vi "FTW-Endpoint-Tell.vi"(0 "FTW Socket":refnum<class "FTW-Endpoint.lvclass">, 5 "Message Header":string, 7 "Message Body":string, 9 "Timeout":i32 format="%dmsec", 11 "error in":errorcluster) -> (4 "FTW Socket out":refnum<class "FTW-Endpoint.lvclass">, 6 "Timed out?":bool, 15 "error out":errorcluster)   [LabVIEW 2012, in "FTW-Actor.lvlib" / "FTW-Endpoint.lvclass"]
uses:
  FTW-Endpoint.lvclass
  Request/FTW-Request.lvclass
panel:
  # "Inputs"
  # "Outputs"
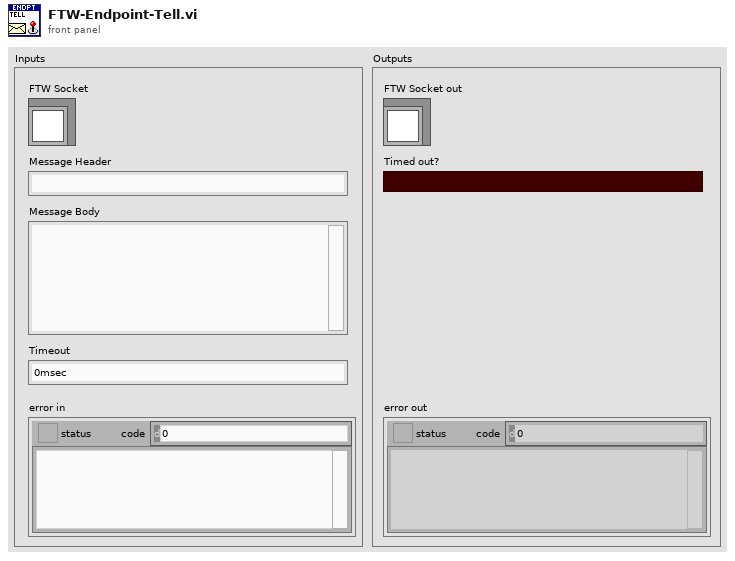
[diagram p1: front panel]
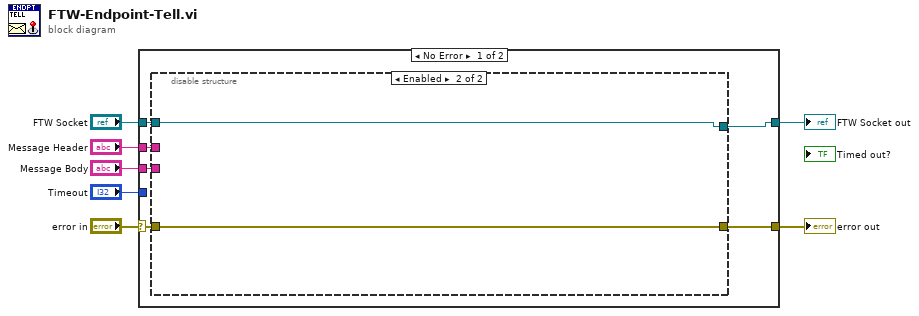
[diagram p0: block diagram]
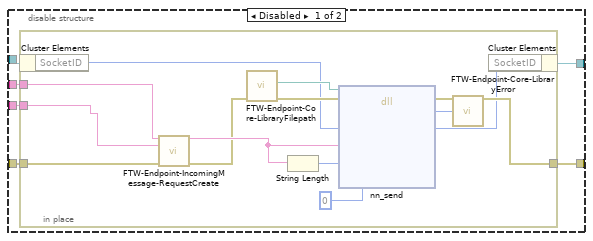
[diagram p2: hidden frame]
diagram:
  n1 = case shown="No Error" "error in" {
    selector: "error in" -> [w11 w37]
    tunnel: [w10 w37] -> w7
    tunnel: [w8 w36] -> w5
    tunnel: "FTW Socket" -> [w9 w36]
    tunnel: "Timeout" -> [_ _]
    tunnel: "Message Header" -> [w13 _]
    tunnel: "Message Body" -> [w12 _]
    frame No Error {
      n2 = disable-structure shown="Enabled" {
        disable-tunnel: w13 -> [w19 _]
        disable-tunnel: w12 -> [w18 _]
        disable-tunnel: w11 -> [w17 w34]
        disable-tunnel: [w16 w34] -> w10
        disable-tunnel: w9 -> [w15 w35]
        disable-tunnel: [w14 w35] -> w8
        frame Disabled {
          n3 = in-place {
            in-place-border: w19 -> [w23]
            in-place-border: w18 -> [w22]
            in-place-border: w17 -> [w24]
            in-place-border: [w27] -> w16
            n4 = in-place-cluster #1(w15) -> ("SocketID"=w26:i64)
            n5 = call "FTW-Endpoint-IncomingMessage-RequestCreate.vi"("Request Header"=w23, "Request Body"=w22, "error in"=w24) -> ("Request"=w21:string, "error out"=w20:errorcluster)  [unwired: 11 in]
            n6 = call "FTW-Endpoint-Core-LibraryFilepath.vi"("error in"=w20) -> ("error out"=w29:errorcluster, "nanomsg Library Filepath"=w28:path)  [unwired: 8 in, 1 out]
            n7 = String Length(string=w21) -> (length=w31:i32)
            n8 = dll-call lib="?" fn="nn_send"(path in=w28, error in=w29, "SocketID"=w26, "Message"=w21, "Message Length"=w31, "Flags"=0) -> (error out=w33:errorcluster, "Return Value"=w32:i64, "SocketID"=w25:i64)  [unwired: 4 in, 1 out]
            n9 = call "FTW-Endpoint-Core-LibraryError.vi"("error in"=w33, "Return Value"=w32) -> ("error out"=w27:errorcluster)  [unwired: 13 in]
            n10 = in-place-cluster #1("SocketID"=w25) -> (w14:refnum<class "FTW-Endpoint.lvclass">)
          }
        }
        frame Enabled {
        }
      }
    }
    frame Error {
    }
  }
  "error out" <- w7
  "FTW Socket out" <- w5
